vi "Gserver_Query.vi"(8 "error in (no error)":errorcluster, 9 "Query":T2, 10 "Requester":string, 11 "FAMM in":refnum<class "FAMM.lvclass">) -> (0 "error out":errorcluster, 3 "FAMM out":refnum<class "FAMM.lvclass">)   [LabVIEW 2020, in "FAMM.lvclass"]
doc: "Andre Koelewijn, 17 jan 2021\n\nThis VI will process a query as received from Gserver,\nthis query is a request for one of the Gviewer instances."
uses:
  FAMM.lvclass
  controls/FAMMrequest.ctl
  Gview/controls/Typedef_Live.ctl
  controls/FAMM_reply_datagram.ctl
  controls/FAMM_reply_PAQdata.ctl
  controls/FAMM_reply_WAQdata.ctl
  controls/FAMM_reply_EAQdata.ctl
  Gserver/controls/Typedef_QueryType.ctl
  FAMM.lvclass/FAMM.ctl
  PAQ-memory.lvclass
  Gview/Gviewer.lvclass
  Gserver/Gserver.lvclass
panel:
  out "T_range":T1
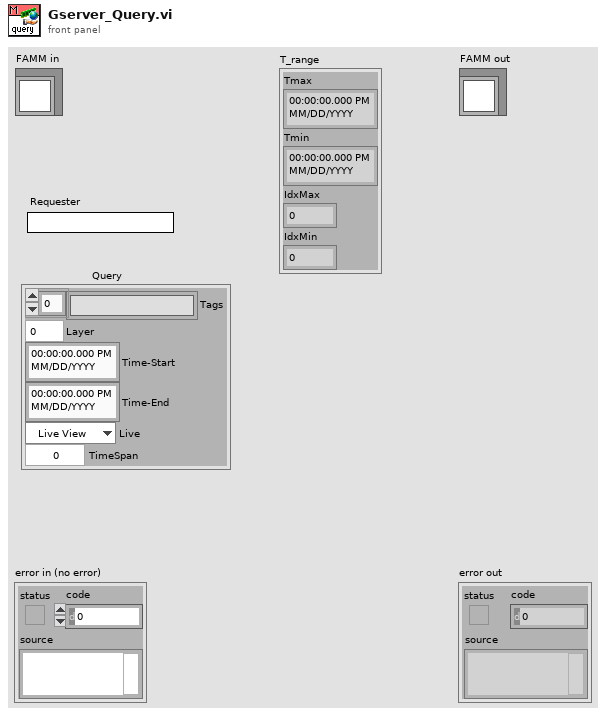
[diagram p1: front panel]
types:
  T1 = cluster{"Tmax":timestamp, "Tmin":timestamp, "IdxMax":i32, "IdxMin":i32}
  T2 = typedef "FAMM.lvclass/FAMMrequest.ctl" = cluster{"Tags":string[], "Layer":i32, "Time-Start":timestamp, "Time-End":timestamp, "Live":T3, "TimeSpan":dbl}
  T3 = typedef "Gviewer.lvclass/Typedef_Live.ctl" = enum16{"Live View", "Freeze"}
  T4 = typedef "Gserver.lvclass/Typedef_QueryType.ctl" = enum16{"Subscribe", "DataRequest", "RequestAllTags", "RequestIniPath", "FAMMstarted", "SetClientOptions", "GviewerUpdate", "OpenNewGraph", "CloseClient", "CloseAllClients", "Close Gserver"}
  T5 = typedef "FAMM.lvclass/FAMM_reply_datagram.ctl" = cluster{"GraphName":string, "Time-Start":timestamp, "Time-End":timestamp, "TimeSpan":dbl, "Live":T3, "PAQ_section":T6, "WAQ_section":T7, "EAQ_section":T8}
  T6 = typedef "FAMM.lvclass/FAMM_reply_PAQdata.ctl" = cluster{"Tags":string[], "time stamp":timestamp[], "DataSection":cluster{"data":dbl[], "max":dbl[], "min":dbl[], "Status":u32[]}[]}
  T7 = typedef "FAMM.lvclass/FAMM_reply_WAQdata.ctl" = cluster{"Boolean":bool}
  T8 = typedef "FAMM.lvclass/FAMM_reply_EAQdata.ctl" = cluster{"Boolean":bool}
  T9 = cluster{"time stamp":timestamp[], "DataSection":cluster{"data":dbl[], "max":dbl[], "min":dbl[], "Status":u32[]}[]}
  T10 = cluster{"data":dbl[], "max":dbl[], "min":dbl[], "Status":u32[]}[]
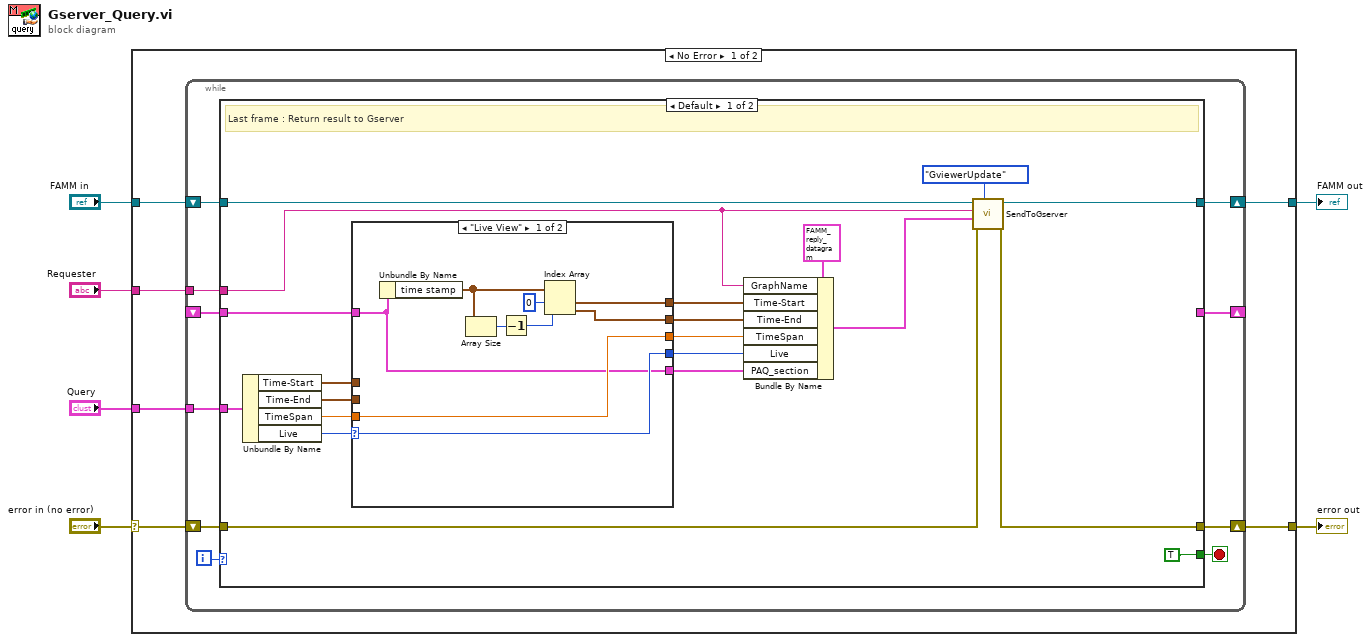
[diagram p0: block diagram]
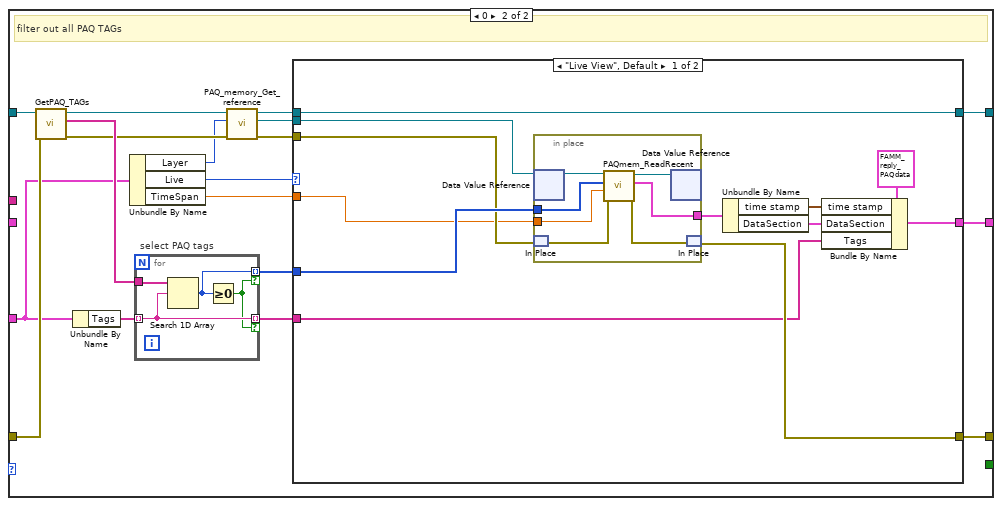
[diagram p3: hidden frame]
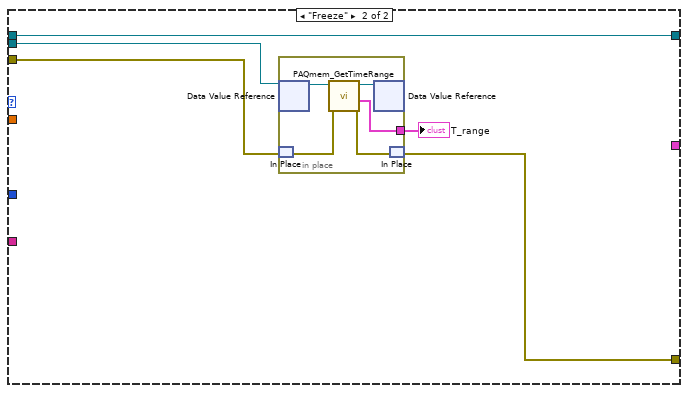
[diagram p4: hidden frame]
diagram:
  n1 = case shown="No Error" "error in (no error)" {
    selector: "error in (no error)" -> [w11 w109]
    tunnel: [w9 w109] -> w5
    tunnel: [w10 w108] -> w3
    tunnel: "FAMM in" -> [w12 w108]
    tunnel: "Requester" -> [w7 _]
    tunnel: "Query" -> [w8 _]
    frame No Error {
      n2 = while {
        shift-right: [w19] -> w10
        shift-left: w12 -> [w20]
        shift-right: [w17] -> w9
        shift-left: w11 -> [w18]
        tunnel: w8 -> [w16]
        shift-right: [w15] -> _
        shift-left: _ -> [w14]
        tunnel: w7 -> [w13]
        i -> [w22]
        stop <- w21 stop-if-true
        n3 = case shown="Default" w22 {
          tunnel: [TRUE _] -> w21
          tunnel: w20 -> [w40 w73]
          tunnel: [w41 w69] -> w19
          tunnel: w18 -> [w38 w71]
          tunnel: [w39 w68] -> w17
          tunnel: w16 -> [w34 w70]
          tunnel: [_ w57] -> w15
          tunnel: w14 -> [w25 _]
          tunnel: w13 -> [w36 _]
          frame Default {
            # "Last frame : Return result to Gserver"
            n4 = Unbundle By Name(w34) -> ("Time-Start"=w29:timestamp, "Time-End"=w27:timestamp, "TimeSpan"=w32:dbl, "Live"=w33:T3)
            n5 = case shown="\"Live View\"" w33 {
              selector: w33 -> [w50 w56]
              tunnel: w32 -> [w51 w55]
              tunnel: [w51 w55] -> w31
              tunnel: [w50 w56] -> w30
              tunnel: w29 -> [_ w54]
              tunnel: [w45 w54] -> w28
              tunnel: w27 -> [_ w53]
              tunnel: [w44 w53] -> w26
              tunnel: w25 -> [w43 w52]
              tunnel: [w43 w52] -> w24
              frame "Live View" {
                n6 = Unbundle By Name(w43) -> ("time stamp"=w49:timestamp[])
                n7 = Array Size(array=w49) -> (size(s)=w47:i32)
                n8 = Decrement(x=w47) -> (x-1=w46:i32)
                n9 = Index Array(array=w49, index #1=0 ("index"), index #2=w46) -> (element #1=w45:timestamp, element #2=w44:timestamp)
              }
              frame "Freeze" {
              }
            }
            n10 = Bundle By Name(cluster=T5 {"GraphName"="", "Time-Start"=timestamp(3693735326.5884657 s since 1904-01-01), "Time-End"=timestamp(3693738926.5884657 s since 1904-01-01), "TimeSpan"=3600.0, "Live"=enum."Live View", "PAQ_section"={"Tags"=[], "time stamp"=[timestamp(3693738906.0787926 s since 1904-01-01), timestamp(3693738907.07885 s since 1904-01-01), timestamp(3693738908.078907 s since 1904-01-01), timestamp(3693738909.0784645 s since 1904-01-01), timestamp(3693738910.078021 s since 1904-01-01), timestamp(3693738911.0780787 s since 1904-01-01), timestamp(3693738912.0781355 s since 1904-01-01), timestamp(3693738913.078193 s since 1904-01-01), timestamp(3693738914.07825 s since 1904-01-01), timestamp(3693738915.078307 s since 1904-01-01), timestamp(3693738916.0783644 s since 1904-01-01), timestamp(3693738917.0784216 s since 1904-01-01), timestamp(3693738918.078479 s since 1904-01-01), timestamp(3693738919.079036 s since 1904-01-01), timestamp(3693738920.0795937 s since 1904-01-01), timestamp(3693738921.079651 s since 1904-01-01), timestamp(3693738922.080208 s since 1904-01-01), timestamp(3693738923.080765 s since 1904-01-01), timestamp(3693738924.080822 s since 1904-01-01), timestamp(3693738925.080879 s since 1904-01-01), timestamp(3693738926.0809364 s since 1904-01-01)], "DataSection"=[{"data"=[0.025001418590545655, 0.025001442432403563, 0.025001442432403563, 0.024976420402526855, 0.025001418590545655, 0.025001442432403563, 0.025001418590545655, 0.025001442432403563, 0.025001418590545655, 0.02500143051147461, 0.02500143051147461, 0.02500143051147461, 0.025001418590545655, 0.025026440620422363, 0.025001442432403563, 0.025001418590545655, 0.025026440620422363, 0.025001418590545655, 0.025001442432403563, 0.025001418590545655, 0.025001442432403563], "max"=[0.025002002716064453, 0.025002002716064453, 0.027001380920410156, 0.025002002716064453, 0.025002002716064453, 0.025002002716064453, 0.025002002716064453, 0.025002002716064453, 0.025002002716064453, 0.025002002716064453, 0.025002002716064453, 0.025002002716064453, 0.025002002716064453, 0.026001453399658203, 0.025002002716064453, 0.025002002716064453, 0.026001930236816406, 0.025002002716064453, 0.025002002716064453, 0.025002002716064453, 0.025002002716064453], "min"=[0.025000572204589844, 0.025000572204589844, 0.023000717163085938, 0.024001598358154297, 0.025000572204589844, 0.025000572204589844, 0.025000572204589844, 0.025000572204589844, 0.025000572204589844, 0.025000572204589844, 0.025000572204589844, 0.025000572204589844, 0.025000572204589844, 0.025000572204589844, 0.025000572204589844, 0.025000572204589844, 0.025000572204589844, 0.025000572204589844, 0.025000572204589844, 0.025000572204589844, 0.025000572204589844], "Status"=[32, 32, 32, 32, 32, 32, 32, 32, 32, 32, 32, 32, 32, 32, 32, 32, 32, 32, 32, 32, 32]}, {"data"=[-0.9354747896064408, -0.8404284269564783, -0.7071607347032589, -0.5418428772577799, -0.35190732133675506, -0.14587999085598086, 0.0667803616892586, 0.2764042621476871, 0.4734603938185778, 0.6489887332802559, 0.7950082939099952, 0.9048796538456292, 0.9736070993342884, 0.9980611009504278, 0.9770997684259897, 0.9117044287198024, 0.804780917615083, 0.6612496881767144, 0.48770429821940564, 0.2919835550131608, 0.08298658586533915], "max"=[-0.8959308174823704, -0.7813847664948913, -0.6313098736866257, -0.45272075499094866, -0.2533811699487135, -0.04252038230785384, 0.1702734124585812, 0.3753254016660106, 0.563311520829305, 0.7256844818543676, 0.8550614257826367, 0.9455595807831805, 0.9930641768448534, 0.9999999409410515, 0.994868561200511, 0.9507995750699587, 0.8634987130737423, 0.736791128791916, 0.5766900244522951, 0.39036772701230454, 0.18629562188798668], "min"=[-0.9684220062635356, -0.8935455880916622, -0.7780405553946977, -0.6271589239650177, -0.44795195781971175, -0.24821082458062316, -0.03718357863555101, 0.17553401560557638, 0.38027060996619916, 0.5677163831595027, 0.7293489873127391, 0.8578186952327538, 0.9472843262210879, 0.993677989367111, 0.9524406630582044, 0.8661801494925992, 0.7403917173979886, 0.5810453180987437, 0.3952793148134019, 0.1915404908565982, -0.02090770788724533], "Status"=[32, 32, 32, 32, 32, 32, 32, 32, 32, 32, 32, 32, 32, 32, 32, 32, 32, 32, 32, 32, 32]}, {"data"=[216.71823637754036, 216.72123654939543, 216.72423687087658, 216.727235467406, 216.73023406403246, 216.73323423540242, 216.73623440725754, 216.73923457862756, 216.74223475041794, 216.74523492182033, 216.74823509364313, 216.75123526514253, 216.75423543673884, 216.75723665836912, 216.76023878024557, 216.76323895158325, 216.76624077346384, 216.76924229486355, 216.77224246675095, 216.77524263812097, 216.77824280984674], "max"=[216.71969896027196, 216.72269913316185, 216.72569930605175, 216.72869647671985, 216.73169664702274, 216.73469681991264, 216.73769699021554, 216.74069716310544, 216.7436973334083, 216.7466975050047, 216.7496976766011, 216.75269784819747, 216.75569801850037, 216.75870119102507, 216.76170136520844, 216.76470153551136, 216.76770470803604, 216.7707048783389, 216.7737050512288, 216.7767052215317, 216.7797053944216], "min"=[216.71677379377394, 216.71977396407684, 216.7227741382602, 216.7257743072696, 216.7287714818182, 216.7317716508276, 216.734771825011, 216.7377719953139, 216.7407721682038, 216.74377233850666, 216.74677251139656, 216.74977268169945, 216.75277285329582, 216.75577302489225, 216.7587761974169, 216.76177636771982, 216.7647765393162, 216.76777971054736, 216.77077988343726, 216.77378005374015, 216.77678022533655], "Status"=[32, 32, 32, 32, 32, 32, 32, 32, 32, 32, 32, 32, 32, 32, 32, 32, 32, 32, 32, 32, 32]}, {"data"=[0.0020000000000000005, 0.0020000000000000005, 0.0020000000000000005, 0.0020000000000000005, 0.0020000000000000005, 0.0020000000000000005, 0.0020000000000000005, 0.0020000000000000005, 0.0020000000000000005, 0.0020000000000000005, 0.0020000000000000005, 0.0020000000000000005, 0.0020000000000000005, 0.0020000000000000005, 0.0020000000000000005, 0.0020000000000000005, 0.0020000000000000005, 0.0020000000000000005, 0.0020000000000000005, 0.0020000000000000005, 0.0020000000000000005], "max"=[0.002, 0.002, 0.002, 0.002, 0.002, 0.002, 0.002, 0.002, 0.002, 0.002, 0.002, 0.002, 0.002, 0.002, 0.002, 0.002, 0.002, 0.002, 0.002, 0.002, 0.002], "min"=[0.002, 0.002, 0.002, 0.002, 0.002, 0.002, 0.002, 0.002, 0.002, 0.002, 0.002, 0.002, 0.002, 0.002, 0.002, 0.002, 0.002, 0.002, 0.002, 0.002, 0.002], "Status"=[32, 32, 32, 32, 32, 32, 32, 32, 32, 32, 32, 32, 32, 32, 32, 32, 32, 32, 32, 32, 32]}, {"data"=[-0.02066160993998472, -0.020661606639795653, -0.02066160333944171, -0.02066160004098581, -0.02066159674252958, -0.02066159344234105, -0.02066159014215198, -0.020661586841963318, -0.020661583541774515, -0.020661580241585716, -0.020661576941396715, -0.020661573641208048, -0.020661570341019446, -0.020661567039675467, -0.02066156373734151, -0.02066156043715298, -0.020661557135149104, -0.02066155383347565, -0.020661550533286516, -0.020661547233097717, -0.020661543932908776], "max"=[-0.020661608331142632, -0.02066160503095477, -0.020661601730764232, -0.0206615984338765, -0.020661595133688627, -0.020661591833498097, -0.020661588533310234, -0.020661585233119697, -0.02066158193293183, -0.02066157863274396, -0.0206615753325561, -0.020661572032365558, -0.020661568732180363, -0.02066156542868969, -0.02066156212849916, -0.02066155882831129, -0.020661555524820626, -0.020661552224632763, -0.020661548924444894, -0.020661545624257028, -0.02066154232406649], "min"=[-0.020661611548827206, -0.020661608248639336, -0.020661604948448806, -0.020661601648260933, -0.020661598351370537, -0.020661595051182664, -0.020661591750992133, -0.02066158845080694, -0.020661585150616397, -0.020661581850428535, -0.020661578550237997, -0.020661575250050135, -0.020661571949862262, -0.02066156864967173, -0.020661565346183727, -0.020661562045995865, -0.020661558745805334, -0.02066155544231733, -0.0206615521421268, -0.02066154884193893, -0.020661545541751064], "Status"=[32, 32, 32, 32, 32, 32, 32, 32, 32, 32, 32, 32, 32, 32, 32, 32, 32, 32, 32, 32, 32]}]}, "WAQ_section"={"Boolean"=FALSE}, "EAQ_section"={"Boolean"=FALSE}} ("GviewerUpdate"), "GraphName"=w36, "Time-Start"=w28, "Time-End"=w26, "TimeSpan"=w31, "Live"=w30, "PAQ_section"=w24) -> (w35:T5)
            n11 = call "SendToGserver.vi"("Query_type"=Typedef_QueryType."GviewerUpdate", "error in (no error)"=w38, "data"=w35, "Address"=w36, "FAMM in"=w40) -> ("error out"=w39:errorcluster, "FAMM out"=w41:refnum<class "FAMM.lvclass">)  [unwired: 5 in]
          }
          frame 0 {
            # "filter out all PAQ TAGs"
            n12 = call "GetPAQ_TAGs.vi"("error in (no error)"=w71, "FAMM in"=w73) -> ("error out"=w64:errorcluster, "PAQ_TAGs"=w72:string[], "FAMM out"=w65:refnum<class "FAMM.lvclass">)  [unwired: 7 in]
            n13 = Unbundle By Name(w70) -> ("Tags"=w74:string[])
            n14 = Unbundle By Name(w70) -> ("Layer"=w63:i32, "Live"=w67:T3, "TimeSpan"=w58:dbl)
            n15 = for "select PAQ tags" {
              tunnel: w74 -> [w106] mode=indexing
              tunnel: w72 -> [w107]
              tunnel: [w106] -> w66 mode=indexing if=w104
              tunnel: [w105] -> w59 mode=indexing if=w104
              n16 = Search 1D Array(1D array=w107, element=w106) -> (index of element=w105:i32)  [unwired: 1 in]
              n17 = Greater Or Equal To 0?(x=w105) -> (x >= 0?=w104:bool)
            }
            n18 = call "PAQ_memory_Get_reference.vi"("error in (no error)"=w64, "PAQ_Layer"=w63, "FAMM in"=w65) -> ("error out"=w61:errorcluster, "PAQ_memory"=w60:refnum<data-value>, "FAMM out"=w62:refnum<class "FAMM.lvclass">)  [unwired: 6 in]
            n19 = case shown="\"Live View\", Default" w67 {
              tunnel: w62 -> [w81 w96]
              tunnel: w61 -> [w83 w95]
              tunnel: [w81 w96] -> w69
              tunnel: [w84 w98] -> w68
              tunnel: w66 -> [w77 _]
              tunnel: w60 -> [w86 w94]
              tunnel: w59 -> [w85 _]
              tunnel: w58 -> [w82 _]
              tunnel: [w76 _] -> w57
              frame "Live View", Default {
                n20 = in-place {
                  in-place-border: w85 -> [w89]
                  in-place-border: w82 -> [w88]
                  in-place-border: [w87] -> w80
                  n21 = in-place-dvr #1(w86) -> (w93:refnum<class "PAQ-memory.lvclass">)  [unwired: 1 out]
                  n22 = in-place-match #2(w83) -> (w91:errorcluster)
                  n23 = call "PAQmem_ReadRecent.vi"("error in (no error)"=w91, "TimeSpan(sec)"=w88, "TagsIndices"=w89, "PAQ-memory in"=w93) -> ("error out"=w90:errorcluster, "PAQ_section"=w87:T9, "PAQ-memory out"=w92:refnum<class "PAQ-memory.lvclass">)  [unwired: 5 in]
                  n24 = in-place-dvr #1(w92) -> ()  [unwired: 2 out]
                  n25 = in-place-match #2(w90) -> (w84:errorcluster)
                }
                n26 = Unbundle By Name(w80) -> ("time stamp"=w79:timestamp[], "DataSection"=w78:T10)
                n27 = Bundle By Name(cluster=T6 {"Tags"=[], "time stamp"=[timestamp(3693738906.0787926 s since 1904-01-01), timestamp(3693738907.07885 s since 1904-01-01), timestamp(3693738908.078907 s since 1904-01-01), timestamp(3693738909.0784645 s since 1904-01-01), timestamp(3693738910.078021 s since 1904-01-01), timestamp(3693738911.0780787 s since 1904-01-01), timestamp(3693738912.0781355 s since 1904-01-01), timestamp(3693738913.078193 s since 1904-01-01), timestamp(3693738914.07825 s since 1904-01-01), timestamp(3693738915.078307 s since 1904-01-01), timestamp(3693738916.0783644 s since 1904-01-01), timestamp(3693738917.0784216 s since 1904-01-01), timestamp(3693738918.078479 s since 1904-01-01), timestamp(3693738919.079036 s since 1904-01-01), timestamp(3693738920.0795937 s since 1904-01-01), timestamp(3693738921.079651 s since 1904-01-01), timestamp(3693738922.080208 s since 1904-01-01), timestamp(3693738923.080765 s since 1904-01-01), timestamp(3693738924.080822 s since 1904-01-01), timestamp(3693738925.080879 s since 1904-01-01), timestamp(3693738926.0809364 s since 1904-01-01)], "DataSection"=[{"data"=[0.025001418590545655, 0.025001442432403563, 0.025001442432403563, 0.024976420402526855, 0.025001418590545655, 0.025001442432403563, 0.025001418590545655, 0.025001442432403563, 0.025001418590545655, 0.02500143051147461, 0.02500143051147461, 0.02500143051147461, 0.025001418590545655, 0.025026440620422363, 0.025001442432403563, 0.025001418590545655, 0.025026440620422363, 0.025001418590545655, 0.025001442432403563, 0.025001418590545655, 0.025001442432403563], "max"=[0.025002002716064453, 0.025002002716064453, 0.027001380920410156, 0.025002002716064453, 0.025002002716064453, 0.025002002716064453, 0.025002002716064453, 0.025002002716064453, 0.025002002716064453, 0.025002002716064453, 0.025002002716064453, 0.025002002716064453, 0.025002002716064453, 0.026001453399658203, 0.025002002716064453, 0.025002002716064453, 0.026001930236816406, 0.025002002716064453, 0.025002002716064453, 0.025002002716064453, 0.025002002716064453], "min"=[0.025000572204589844, 0.025000572204589844, 0.023000717163085938, 0.024001598358154297, 0.025000572204589844, 0.025000572204589844, 0.025000572204589844, 0.025000572204589844, 0.025000572204589844, 0.025000572204589844, 0.025000572204589844, 0.025000572204589844, 0.025000572204589844, 0.025000572204589844, 0.025000572204589844, 0.025000572204589844, 0.025000572204589844, 0.025000572204589844, 0.025000572204589844, 0.025000572204589844, 0.025000572204589844], "Status"=[32, 32, 32, 32, 32, 32, 32, 32, 32, 32, 32, 32, 32, 32, 32, 32, 32, 32, 32, 32, 32]}, {"data"=[-0.9354747896064408, -0.8404284269564783, -0.7071607347032589, -0.5418428772577799, -0.35190732133675506, -0.14587999085598086, 0.0667803616892586, 0.2764042621476871, 0.4734603938185778, 0.6489887332802559, 0.7950082939099952, 0.9048796538456292, 0.9736070993342884, 0.9980611009504278, 0.9770997684259897, 0.9117044287198024, 0.804780917615083, 0.6612496881767144, 0.48770429821940564, 0.2919835550131608, 0.08298658586533915], "max"=[-0.8959308174823704, -0.7813847664948913, -0.6313098736866257, -0.45272075499094866, -0.2533811699487135, -0.04252038230785384, 0.1702734124585812, 0.3753254016660106, 0.563311520829305, 0.7256844818543676, 0.8550614257826367, 0.9455595807831805, 0.9930641768448534, 0.9999999409410515, 0.994868561200511, 0.9507995750699587, 0.8634987130737423, 0.736791128791916, 0.5766900244522951, 0.39036772701230454, 0.18629562188798668], "min"=[-0.9684220062635356, -0.8935455880916622, -0.7780405553946977, -0.6271589239650177, -0.44795195781971175, -0.24821082458062316, -0.03718357863555101, 0.17553401560557638, 0.38027060996619916, 0.5677163831595027, 0.7293489873127391, 0.8578186952327538, 0.9472843262210879, 0.993677989367111, 0.9524406630582044, 0.8661801494925992, 0.7403917173979886, 0.5810453180987437, 0.3952793148134019, 0.1915404908565982, -0.02090770788724533], "Status"=[32, 32, 32, 32, 32, 32, 32, 32, 32, 32, 32, 32, 32, 32, 32, 32, 32, 32, 32, 32, 32]}, {"data"=[216.71823637754036, 216.72123654939543, 216.72423687087658, 216.727235467406, 216.73023406403246, 216.73323423540242, 216.73623440725754, 216.73923457862756, 216.74223475041794, 216.74523492182033, 216.74823509364313, 216.75123526514253, 216.75423543673884, 216.75723665836912, 216.76023878024557, 216.76323895158325, 216.76624077346384, 216.76924229486355, 216.77224246675095, 216.77524263812097, 216.77824280984674], "max"=[216.71969896027196, 216.72269913316185, 216.72569930605175, 216.72869647671985, 216.73169664702274, 216.73469681991264, 216.73769699021554, 216.74069716310544, 216.7436973334083, 216.7466975050047, 216.7496976766011, 216.75269784819747, 216.75569801850037, 216.75870119102507, 216.76170136520844, 216.76470153551136, 216.76770470803604, 216.7707048783389, 216.7737050512288, 216.7767052215317, 216.7797053944216], "min"=[216.71677379377394, 216.71977396407684, 216.7227741382602, 216.7257743072696, 216.7287714818182, 216.7317716508276, 216.734771825011, 216.7377719953139, 216.7407721682038, 216.74377233850666, 216.74677251139656, 216.74977268169945, 216.75277285329582, 216.75577302489225, 216.7587761974169, 216.76177636771982, 216.7647765393162, 216.76777971054736, 216.77077988343726, 216.77378005374015, 216.77678022533655], "Status"=[32, 32, 32, 32, 32, 32, 32, 32, 32, 32, 32, 32, 32, 32, 32, 32, 32, 32, 32, 32, 32]}, {"data"=[0.0020000000000000005, 0.0020000000000000005, 0.0020000000000000005, 0.0020000000000000005, 0.0020000000000000005, 0.0020000000000000005, 0.0020000000000000005, 0.0020000000000000005, 0.0020000000000000005, 0.0020000000000000005, 0.0020000000000000005, 0.0020000000000000005, 0.0020000000000000005, 0.0020000000000000005, 0.0020000000000000005, 0.0020000000000000005, 0.0020000000000000005, 0.0020000000000000005, 0.0020000000000000005, 0.0020000000000000005, 0.0020000000000000005], "max"=[0.002, 0.002, 0.002, 0.002, 0.002, 0.002, 0.002, 0.002, 0.002, 0.002, 0.002, 0.002, 0.002, 0.002, 0.002, 0.002, 0.002, 0.002, 0.002, 0.002, 0.002], "min"=[0.002, 0.002, 0.002, 0.002, 0.002, 0.002, 0.002, 0.002, 0.002, 0.002, 0.002, 0.002, 0.002, 0.002, 0.002, 0.002, 0.002, 0.002, 0.002, 0.002, 0.002], "Status"=[32, 32, 32, 32, 32, 32, 32, 32, 32, 32, 32, 32, 32, 32, 32, 32, 32, 32, 32, 32, 32]}, {"data"=[-0.02066160993998472, -0.020661606639795653, -0.02066160333944171, -0.02066160004098581, -0.02066159674252958, -0.02066159344234105, -0.02066159014215198, -0.020661586841963318, -0.020661583541774515, -0.020661580241585716, -0.020661576941396715, -0.020661573641208048, -0.020661570341019446, -0.020661567039675467, -0.02066156373734151, -0.02066156043715298, -0.020661557135149104, -0.02066155383347565, -0.020661550533286516, -0.020661547233097717, -0.020661543932908776], "max"=[-0.020661608331142632, -0.02066160503095477, -0.020661601730764232, -0.0206615984338765, -0.020661595133688627, -0.020661591833498097, -0.020661588533310234, -0.020661585233119697, -0.02066158193293183, -0.02066157863274396, -0.0206615753325561, -0.020661572032365558, -0.020661568732180363, -0.02066156542868969, -0.02066156212849916, -0.02066155882831129, -0.020661555524820626, -0.020661552224632763, -0.020661548924444894, -0.020661545624257028, -0.02066154232406649], "min"=[-0.020661611548827206, -0.020661608248639336, -0.020661604948448806, -0.020661601648260933, -0.020661598351370537, -0.020661595051182664, -0.020661591750992133, -0.02066158845080694, -0.020661585150616397, -0.020661581850428535, -0.020661578550237997, -0.020661575250050135, -0.020661571949862262, -0.02066156864967173, -0.020661565346183727, -0.020661562045995865, -0.020661558745805334, -0.02066155544231733, -0.0206615521421268, -0.02066154884193893, -0.020661545541751064], "Status"=[32, 32, 32, 32, 32, 32, 32, 32, 32, 32, 32, 32, 32, 32, 32, 32, 32, 32, 32, 32, 32]}]} ("PAQ_section"), "time stamp"=w79, "DataSection"=w78, "Tags"=w77) -> (w76:T6)
              }
              frame "Freeze" {
                n28 = in-place {
                  in-place-border: [w99] -> w97
                  n29 = in-place-dvr #3(w94) -> (w103:refnum<class "PAQ-memory.lvclass">)  [unwired: 1 out]
                  n30 = in-place-match #4(w95) -> (w100:errorcluster)
                  n31 = call "PAQmem_GetTimeRange.vi"("error in (no error)"=w100, "PAQ-memory in"=w103) -> ("error out"=w101:errorcluster, "T_range"=w99:T1, "PAQ-memory out"=w102:refnum<class "PAQ-memory.lvclass">)  [unwired: 7 in]
                  n32 = in-place-dvr #3(w102) -> ()  [unwired: 2 out]
                  n33 = in-place-match #4(w101) -> (w98:errorcluster)
                }
                "T_range" <- w97
              }
            }
          }
        }
      }
    }
    frame Error {
    }
  }
  "error out" <- w5
  "FAMM out" <- w3
